vi "read-stoil.vi"(11 "file path (use dialog)":path=path "C:/Users/lsv/Documents/Sys/AVIA/AI-04/speed/VI/STOIL.FOR") -> (0 "ACPS":dbl[](array[numeric]), 1 "AS":dbl[](array[numeric]), 2 "ACPH":dbl[](array[numeric]), 3 "AH":dbl[](array[numeric]))   [LabVIEW 2011]
doc: "read STOIL for MAX calculation"
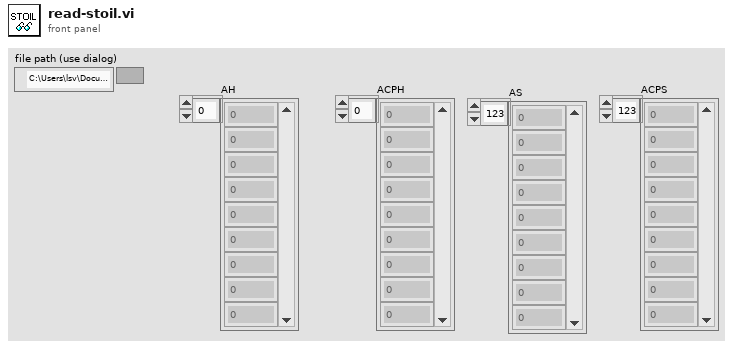
[diagram p1: front panel]
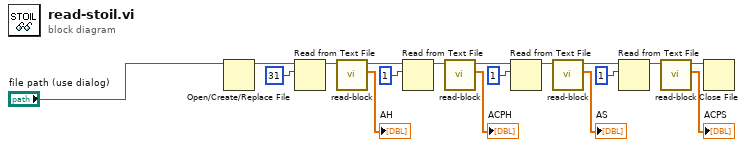
[diagram p0: block diagram]
diagram:
  n1 = Open/Create/Replace File(file path (use dialog)="file path (use dialog)") -> (refnum out=w18:refnum<file>)  [unwired: 5 in, 2 out]
  n2 = Read from Text File(file (use dialog)=w18, count=31) -> (refnum out=w17:refnum<file>)  [unwired: 2 in, 3 out]
  n3 = call "read-block.vi"("Byte Stream File in"=w17) -> ("Array"=→"AH":dbl[], "Byte Stream File out"=w13:refnum<file>)  [unwired: 9 in]
  n4 = Read from Text File(file (use dialog)=w13, count=1) -> (refnum out=w11:refnum<file>)  [unwired: 2 in, 3 out]
  n5 = call "read-block.vi"("Byte Stream File in"=w11) -> ("Array"=→"ACPH":dbl[], "Byte Stream File out"=w5:refnum<file>)  [unwired: 9 in]
  n6 = Read from Text File(file (use dialog)=w5, count=1) -> (refnum out=w9:refnum<file>)  [unwired: 2 in, 3 out]
  n7 = call "read-block.vi"("Byte Stream File in"=w9) -> ("Array"=→"AS":dbl[], "Byte Stream File out"=w4:refnum<file>)  [unwired: 9 in]
  n8 = Read from Text File(file (use dialog)=w4, count=1) -> (refnum out=w6:refnum<file>)  [unwired: 2 in, 3 out]
  n9 = call "read-block.vi"("Byte Stream File in"=w6) -> ("Array"=→"ACPS":dbl[], "Byte Stream File out"=w3:refnum<file>)  [unwired: 9 in]
  n10 = Close File(refnum=w3) -> ()  [unwired: 1 in, 2 out]
